vi "TCE_Config_Save.vi"(8 "error in":errorcluster, 11 "Config":T1={"Freezing"={"Cutoff"=2.0, "EndIndex"=2}}) -> (0 "error out":errorcluster, 3 "Config dup":T1={"Freezing"={"Cutoff"=2.0, "EndIndex"=2}})   [LabVIEW 2022 SP3]
uses:
  TCE_Config.ctl
  <vilib>/Utility/xml.llb/Write to XML File(string).vi
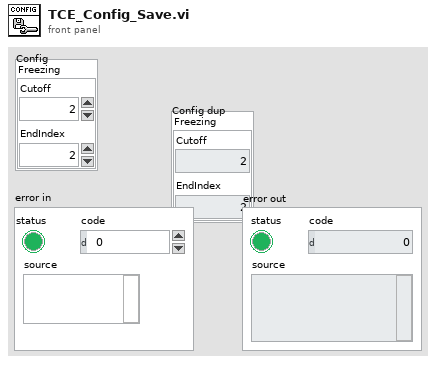
[diagram p1: front panel]
types:
  T1 = typedef "TCE_Config.ctl" = cluster{"Freezing":cluster{"Cutoff":dbl, "EndIndex":i32}}
  T2 = enum16{"open", "replace", "create", "open or create", "replace or create", "replace or create with confirmation"}
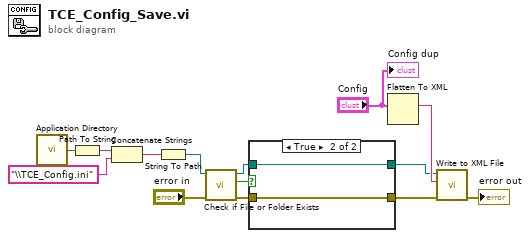
[diagram p0: block diagram]
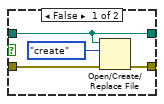
[diagram p2: hidden frame]
diagram:
  n1 = call <vilib>:"Application Directory.vi"() -> ("Application Directory"=w12:path)
  n2 = Path To String(path=w12) -> (string=w13:string)
  n3 = Concatenate Strings(w13, "\\TCE_Config.ini" ("string")) -> (w10:string)
  n4 = String To Path(string=w10) -> (path=w9:path)
  n5 = call <vilib>:"Check if File or Folder Exists.vi"("error in (no error)"="error in", "path"=w9) -> ("error out"=w6:errorcluster, "file or folder exists?"=w8:bool, "dup path"=w7:path)  [unwired: 7 in]
  n6 = case shown="True" w8 {
    tunnel: w7 -> [w15 w19]
    tunnel: w6 -> [w17 w20]
    tunnel: [w16 w20] -> w5
    tunnel: [w15 w19] -> w4
    frame False {
      n7 = Open/Create/Replace File(file path (use dialog)=w15, error in=w17, operation (0:open)=T2."create") -> (error out=w16:errorcluster)  [unwired: 3 in, 2 out]
    }
    frame True {
    }
  }
  n8 = Flatten To XML(6:"Config") -> (2:w14:string)
  n9 = call-poly <vilib>:"Write to XML File.vi"("error in (no error)"=w5, "XML Input"=w14, "XML File Path"=w4) -> ("error out"=→"error out":errorcluster)  [unwired: 6 in, 2 out]
  "Config dup" <- "Config"
